vi "_digital_on_duration_off.vi"(10 "duration (ms)":dbl=20.0, 11 "digital port":tag="Dev1/port1/line2") -> ()   [LabVIEW 2010]
uses:
  <vilib>/DAQmx/write.llb/DAQmx Write (Digital Bool 1Line 1Point).vi
  <vilib>/DAQmx/create/channels.llb/DAQmx Create Channel (DO-Digital Output).vi
  <vilib>/daqmx/miscellaneous.llb/DAQmx Fill In Error Info.vi
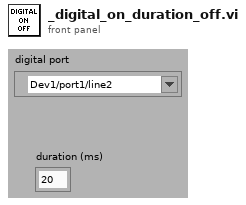
[diagram p1: front panel]
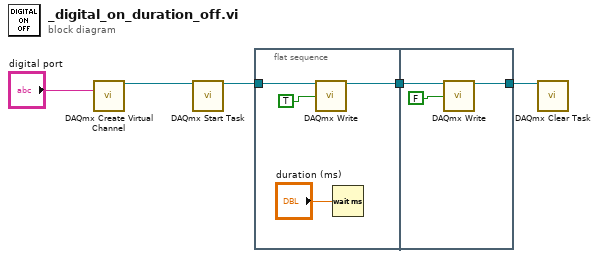
[diagram p0: block diagram]
diagram:
  n1 = call-poly <vilib>:"DAQmx Create Virtual Channel.vi"("lines"="digital port") -> ("task out"=w4:refnum<k21>)  [unwired: 13 in, 1 out]
  n2 = call <vilib>:"DAQmx Start Task.vi"("task/channels in"=w4) -> ("task out"=w3:refnum<k21>)  [unwired: 13 in, 1 out]
  n3 = flat-sequence {
    tunnel: w3 -> [w9]
    tunnel: [w7] -> w2
    tunnel: w2 -> [w12]
    tunnel: [w11] -> w1
    frame #0 {
      n4 = call-poly <vilib>:"DAQmx Write.vi"("task/channels in"=w9, "data"=TRUE) -> ("task out"=w7:refnum<k21>)  [unwired: 11 in, 2 out]
      n5 = Wait (ms)(milliseconds to wait="duration (ms)") -> ()  [unwired: 1 out]
    }
    frame #1 {
      n6 = call-poly <vilib>:"DAQmx Write.vi"("task/channels in"=w12, "data"=FALSE) -> ("task out"=w11:refnum<k21>)  [unwired: 11 in, 2 out]
    }
  }
  n7 = call <vilib>:"DAQmx Clear Task.vi"("task in"=w1) -> ()  [unwired: 14 in, 1 out]
